vi "HackRF_Write_Int8.vi"(8 "error in (no error)":errorcluster, 9 "Q data":i8[](array[numeric]), 10 "I data":i8[](array[numeric]), 11 "HackRF":T1) -> (0 "error out":errorcluster, 3 "HackRF":T1)   [LabVIEW 2020]
uses:
  HackRF_Ref.ctl
  D:/Programming/Labview/HackRF/HackRF_Lib/NetHackrf.dll
  NetHackrf.dll
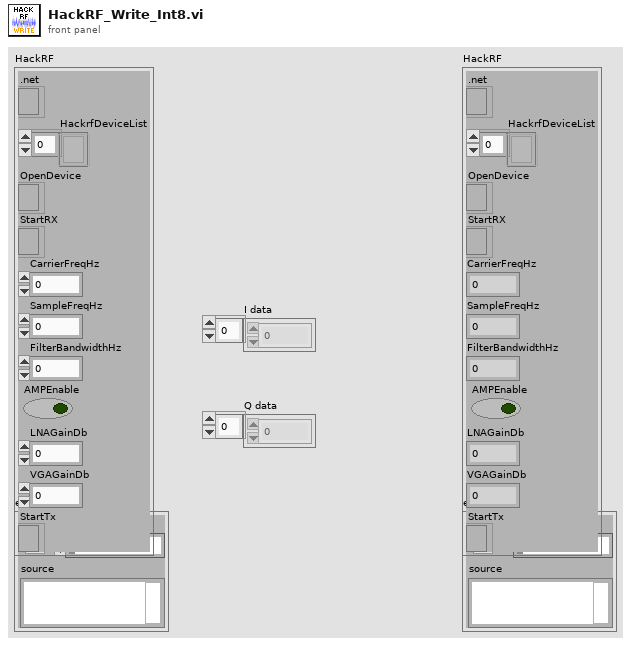
[diagram p1: front panel]
types:
  T1 = typedef "HackRF_Ref.ctl" = cluster{".net":refnum<k24>, "HackrfDeviceList":refnum<k24>[], "OpenDevice":refnum<k24>, "StartRX":refnum<k24>, "CarrierFreqHz":dbl, "SampleFreqHz":dbl, "FilterBandwidthHz":dbl, "AMPEnable":bool, "LNAGainDb":dbl, "VGAGainDb":dbl, "StartTx":refnum<k24>}
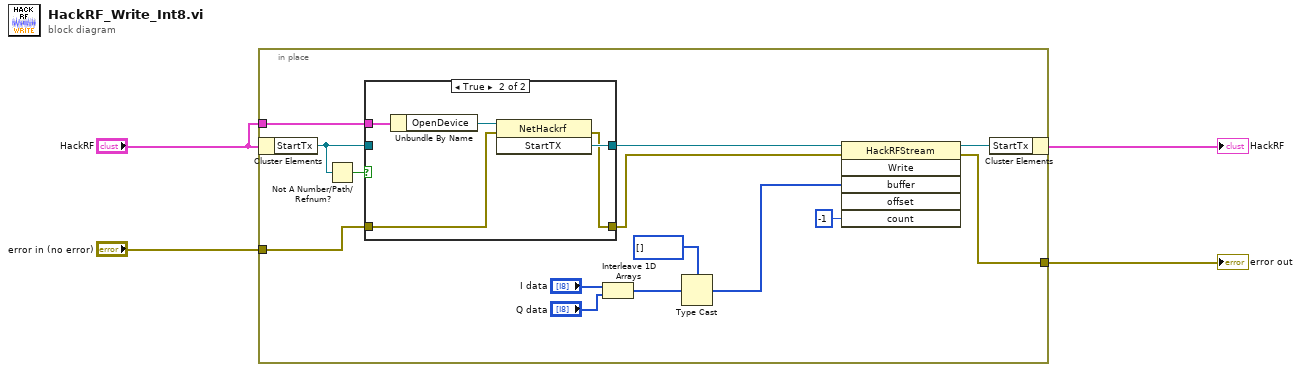
[diagram p0: block diagram]
diagram:
  n1 = in-place {
    in-place-border: "HackRF" -> [w17]
    in-place-border: "error in (no error)" -> [w15]
    in-place-border: [w13] -> w4
    n2 = in-place-cluster #1("HackRF") -> ("StartTx"=w16:refnum<k24>)
    n3 = Not A Number/Path/Refnum?(number/path/refnum=w16) -> (NaN/Path/Refnum?=w18:bool)
    n4 = case shown="True" w18 {
      tunnel: [w20 w25] -> w11
      tunnel: w17 -> [_ w24]
      tunnel: w16 -> [w20 _]
      tunnel: w15 -> [w19 w21]
      tunnel: [w19 w22] -> w14
      frame False {
      }
      frame True {
        n5 = Unbundle By Name(w24) -> ("OpenDevice"=w23:refnum<k24>)
        n6 = invoke class="NetHackrf" method="StartTX"(reference=w23, error in=w21) -> (error out=w22:errorcluster, "StartTX"=w25:refnum<k24>)  [unwired: 1 in, 1 out]
      }
    }
    n7 = Interleave 1D Arrays("I data", "Q data") -> (w6:i8[])
    n8 = Type Cast(type=i8[] [] ("8bit integer"), x=w6) -> (*(type *) &x=w5:i8[])
    n9 = invoke class="HackRFStream" method="Write"(reference=w11, error in=w14, "buffer"=w5, "count"=-1) -> (reference out=w12:refnum<k24>, error out=w13:errorcluster)  [unwired: 2 in, 4 out]
    n10 = in-place-cluster #1("StartTx"=w12) -> (→"HackRF":T1)
  }
  "error out" <- w4
